vi "Record.vi"(9 "stop (F)":bool, 10 "Seconds to Record":dbl, 11 "file path (dialog if empty)":path) -> (2 "Recorded Signal":dynamicdata(graph))   [LabVIEW 2014]
uses:
  <vilib>/Waveform/WDTFileIO.llb/ Write Waveforms to File (1D).vi
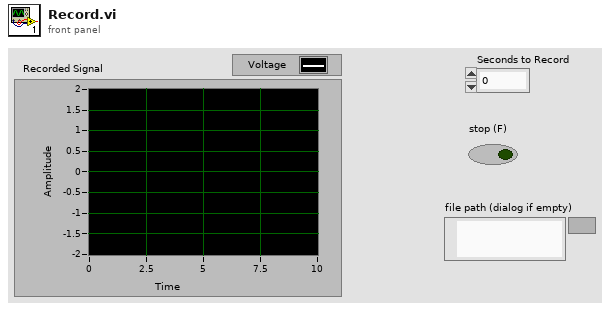
[diagram p1: front panel]
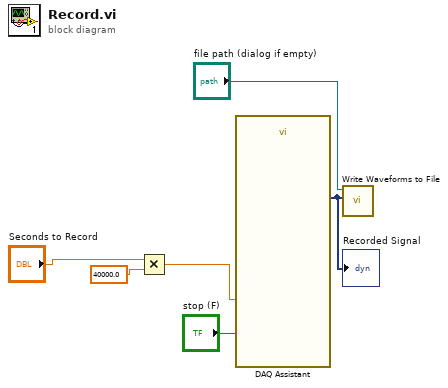
[diagram p0: block diagram]
diagram:
  n1 = Multiply(x="Seconds to Record", y=40000.0) -> (x*y=w1:dbl)
  n2 = call "DAQ Assistant"("number of samples"=w1, "stop (F)"="stop (F)") -> ("data"=w6:dynamicdata)  [unwired: 14 in, 3 out]
  "Recorded Signal" <- w6
  n3 = call-poly <vilib>:"Write Waveforms to File.vi"("waveform array"=w6, "file path (dialog if empty)"="file path (dialog if empty)") -> ()  [unwired: 8 in, 2 out]
